vi "DO Remains.vi"(11 "Array":T1(array[cluster])) -> (1 "DO value":bool[](array[boolean]), 2 "Same DO":T1(array[cluster]), 3 "Remains":T1(array[cluster]))   [LabVIEW 2022 SP3]
panel:
  in  "Read DO":bool[](array[boolean])=[FALSE, FALSE, TRUE, FALSE, FALSE, FALSE, FALSE, FALSE]
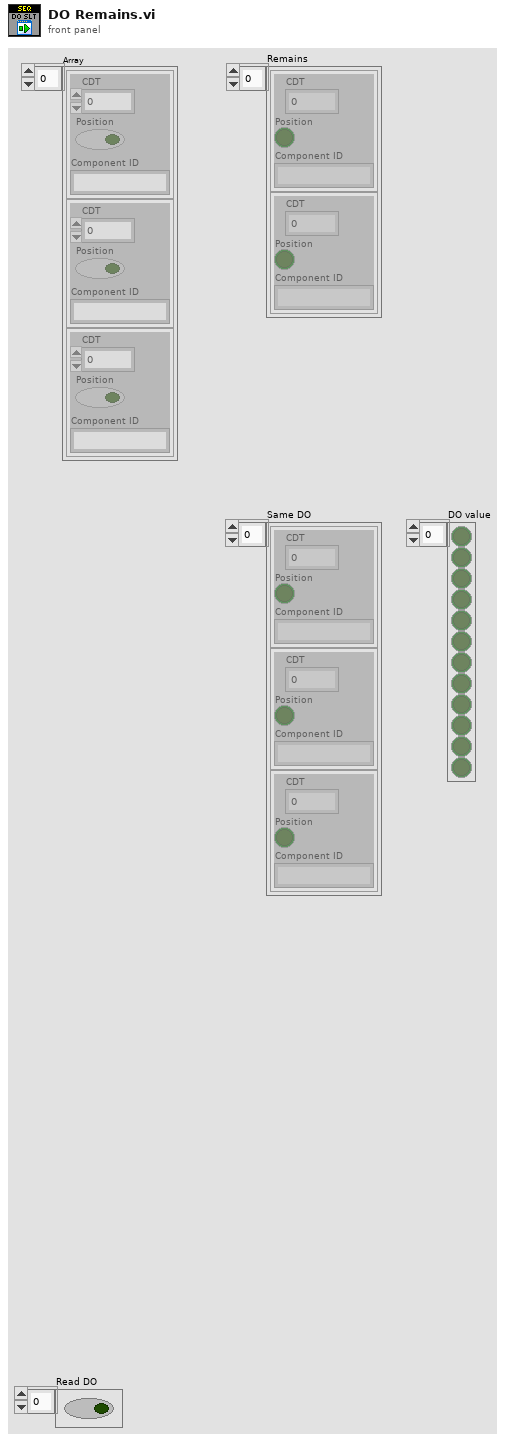
[diagram p1: front panel]
types:
  T1 = cluster{"CDT":dbl, "Position":bool, "Component ID":string}[]
  T2 = cluster{"CDT":dbl, "Position":bool, "Component ID":string}
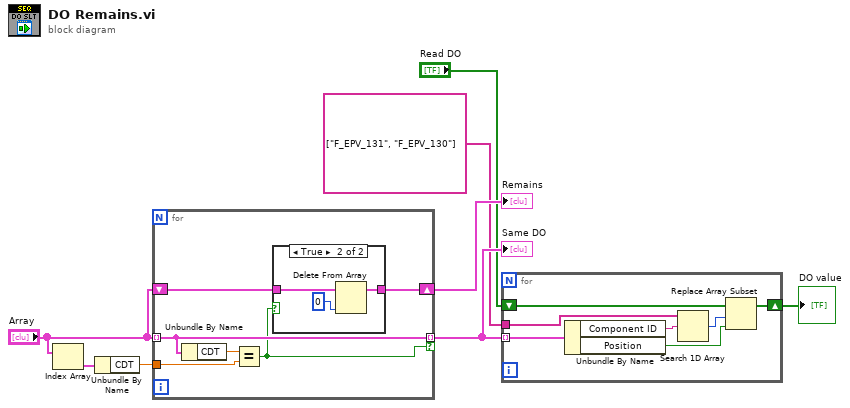
[diagram p0: block diagram]
diagram:
  n1 = Index Array(array="Array") -> (element=w5:T2)  [unwired: 1 in]
  n2 = Unbundle By Name(w5) -> ("CDT"=w7:dbl)
  n3 = for {
    tunnel: "Array" -> [w10] mode=indexing
    shift-right: [w13] -> w8
    shift-left: "Array" -> [w14]
    tunnel: w7 -> [w11]
    tunnel: [w10] -> w4 mode=indexing if=w9
    n4 = Unbundle By Name(w10) -> ("CDT"=w12:dbl)
    n5 = Equal?(x=w12, y=w11) -> (x = y?=w9:bool)
    n6 = case shown="True" w9 {
      tunnel: w14 -> [w15 w18]
      tunnel: [w15 w17] -> w13
      frame False {
      }
      frame True {
        n7 = Delete From Array(array=w18, index=0) -> (array with subset deleted=w17:T1)  [unwired: 1 in, 1 out]
      }
    }
  }
  "Remains" <- w8
  "Same DO" <- w4
  n8 = for {
    tunnel: w4 -> [w25] mode=indexing
    tunnel: string[] ["F_EPV_131", "F_EPV_130"] -> [w24]
    shift-right: [w19] -> w1
    shift-left: "Read DO" -> [w23]
    n9 = Unbundle By Name(w25) -> ("Component ID"=w21:string, "Position"=w20:bool)
    n10 = Search 1D Array(1D array=w24, element=w21) -> (index of element=w22:i32)  [unwired: 1 in]
    n11 = Replace Array Subset(array=w23, new element=w20, index=w22) -> (w19:bool[])
  }
  "DO value" <- w1
